vi "Parse Opcode.vi"(8 "error in":errorcluster, 11 "Opcode":string) -> (0 "Error out":errorcluster, 3 "Opcode Array":string[](array[string]))   [LabVIEW 2018, in "File Parser Interface.lvlib" / "File Parser Interface.lvclass"]
uses:
  File Parser Interface.lvclass
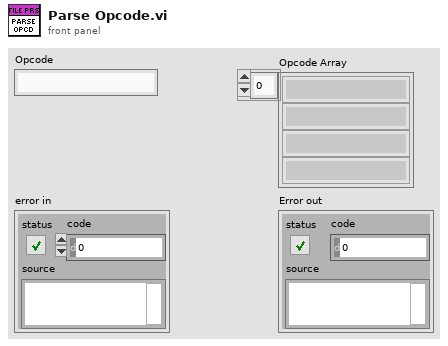
[diagram p1: front panel]
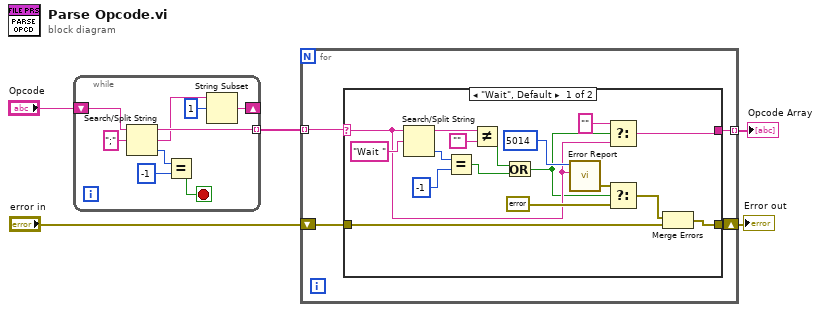
[diagram p0: block diagram]
diagram:
  n1 = while {
    shift-right: [w8] -> _
    shift-left: "Opcode" -> [w13]
    tunnel: [w9] -> w3 mode=indexing
    stop <- w10 stop-if-true
    n2 = Search/Split String(string=w13, search string/char (-)=";") -> (substring before match=w9:string, match + rest of string=w7:string, offset of match=w12:i32)  [unwired: 1 in]
    n3 = Equal?(x=w12, y=-1) -> (x = y?=w10:bool)
    n4 = String Subset(string=w7, offset (0)=1) -> (substring=w8:string)  [unwired: 1 in]
  }
  n5 = for {
    shift-right: [w18] -> w5
    shift-left: "error in" -> [w16]
    tunnel: w3 -> [w17] mode=indexing
    tunnel: [w15] -> w1 mode=indexing
    n6 = case shown="\"Wait\", Default" w17 {
      selector: w17 -> [w24 w37]
      tunnel: [w25 w36] -> w18
      tunnel: [w29 w37] -> w15
      tunnel: w16 -> [w26 w36]
      frame "Wait", Default {
        n7 = Search/Split String(string=w24, search string/char (-)="Wait " ("search string")) -> (substring before match=w23:string, offset of match=w34:i32)  [unwired: 1 in, 1 out]
        n8 = Equal?(x=w34, y=-1) -> (x = y?=w20:bool)
        n9 = Not Equal?(x=w23, y="") -> (x != y?=w21:bool)
        n10 = Or(x=w21, y=w20) -> (x .or. y?=w19:bool)
        n11 = call "Error Report.vi"("Additional info"=w24, "Error Code"=i16 5014) -> ("error out"=w31:errorcluster)  [unwired: 9 in]
        n12 = Select(t="", s=w19, f=w24) -> (s? t:f=w29:string)
        n13 = Select(t=w31, s=w19, f=errorcluster {"status"=FALSE, "code"=0, "source"=""}) -> (s? t:f=w27:errorcluster)
        n14 = Merge Errors(w27, w26) -> (w25:errorcluster)
      }
      frame "", "First", "Last", "Trig", "pulse_signal(event0)" {
      }
    }
  }
  "Error out" <- w5
  "Opcode Array" <- w1
